vi "Batch property change.vi"   [LabVIEW 2017]
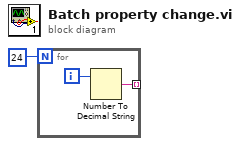
[diagram p0: block diagram]
diagram:
  n1 = for {
    N: 24 -> [_]
    tunnel: [w2] -> _ mode=indexing
    i -> [w3]
    n2 = Number To Decimal String(number=w3) -> (decimal integer string=w2:string)  [unwired: 1 in]
  }
